vi "Destroy.vi"(8 "error in (no error)":errorcluster, 11 "LinkedEventMessenger in":refnum<class "LinkedEventMessenger.lvclass">) -> (0 "error out":errorcluster)   [LabVIEW 2011, in "Messenging.lvlib" / "LinkedEventMessenger.lvclass"]
uses:
  LinkedEventMessenger.lvclass
  LinkedEventMessenger.lvclass/LinkedEventMessenger.ctl
  Messenger (Parent)/MGR.lvclass
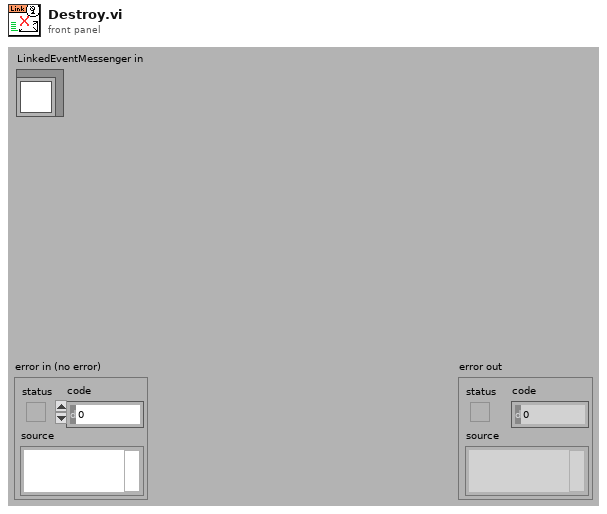
[diagram p1: front panel]
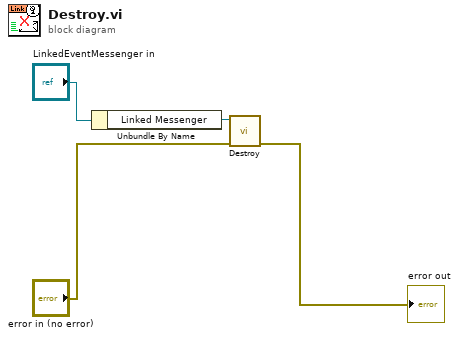
[diagram p0: block diagram]
diagram:
  n1 = Unbundle By Name("LinkedEventMessenger in") -> ("Linked Messenger"=w3:refnum<class "MGR.lvclass">)
  n2 = call-dynamic "Destroy.vi"("error in (no error)"="error in (no error)", "Messenger in"=w3) -> ("error out"=→"error out":errorcluster)  [unwired: 9 out]
